vi "Cap_Input.vi"(4 "error in (no error)":errorcluster, 5 "Measured origin x,y":dbl[](array[numeric])=[0.83, 0.79], 6 "Element In":T3, 7 "Outputmode":u16(ring) items=["Get Path", "Make Layout", "Create TRJs"]) -> (0 "error out":errorcluster, 1 "Init Cluster":T6, 2 "TRJs":T4, 3 "Elements Out":T5(array[cluster]))   [LabVIEW 2009]
panel:
  out "output cluster":T1
  in  "Tab Control":enum32{"Main", "Expert", "Output"}(tab)=enum."Output"
  in  "Length of Cap":dbl=3.0
  in  "Radus of Cap":dbl=0.1
  in  "Ab rate":dbl=0.005
  in  "Interval of  laser path":dbl=0.008
  in  "Height to cap":dbl=3.0
  in  "stop":bool
  in  "XY Line Arc Trajectory part 1":T2={"Velocity (units/s)"=2.0, "Acceleration (unts/s2)"=20.0, "Number of times of execution"=1} {"Acceleration (unts/s2)" format="%.6f"; "Velocity (units/s)" format="%.6f"; "Number of times of execution" format="%.6f"}
  in  "Type":i32
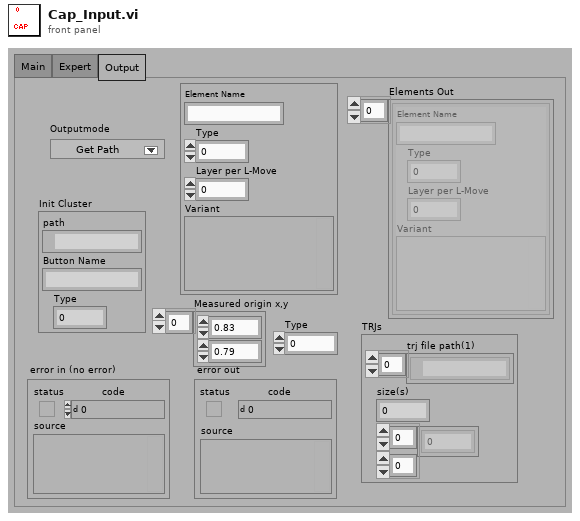
[diagram p1: front panel]
types:
  T1 = cluster{"Length of Cap":dbl, "Height to cap":dbl, "Radus of Cap ":dbl, "Ab rate":dbl, "Interval of  laser path":dbl, "Velocity (units/s)":dbl, "Acceleration (unts/s2)":dbl, "Number of times of execution":i32}
  T2 = cluster{"Velocity (units/s)":dbl, "Acceleration (unts/s2)":dbl, "Number of times of execution":i32}
  T3 = cluster{"Element Name":string, "Type":i32, "Layer per L-Move":i32, "Variant":variant}
  T4 = cluster{"trj file path(1)":path[], "size(s)":i32, dbl[][]}
  T5 = cluster{"Element Name":string, "Type":i32, "Layer per L-Move":i32, "Variant":variant}[]
  T6 = cluster{"path":path, "Button Name":string, "Type":i32}
  T7 = cluster{"Element Name":string, "Value":i32, "Layer per L-Move":i32, "Variant":variant}
  T8 = cluster{"Element Name":string, "Value":i32, "Layer per L-Move":i32, "Variant":variant}[]
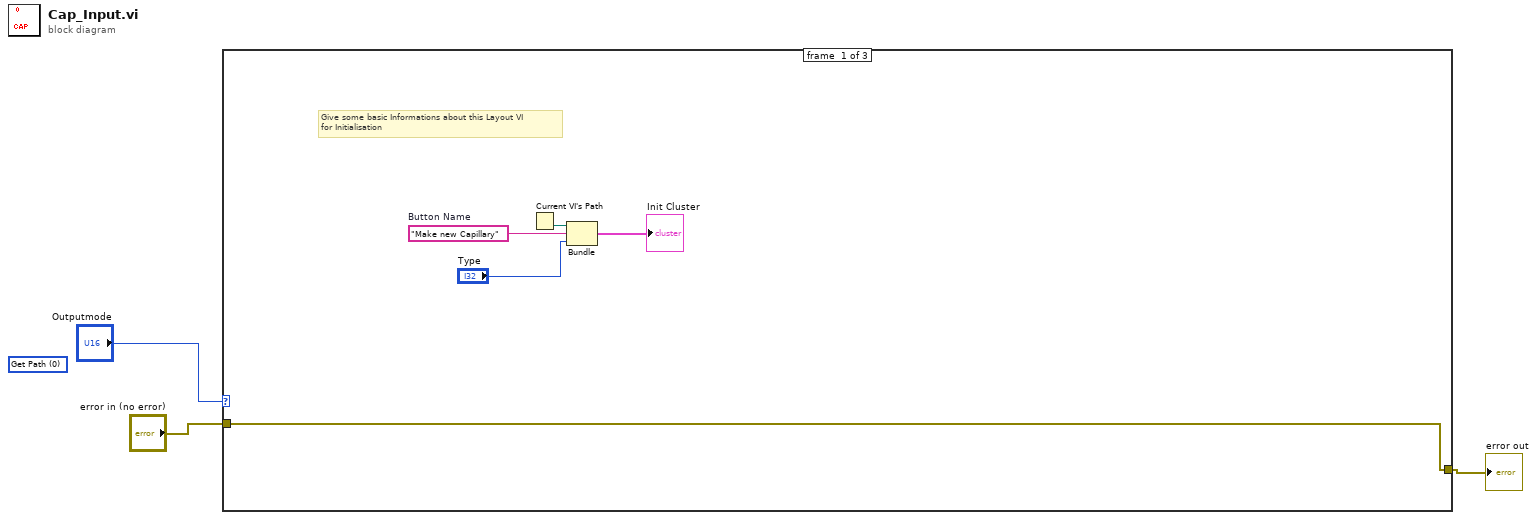
[diagram p0: block diagram]
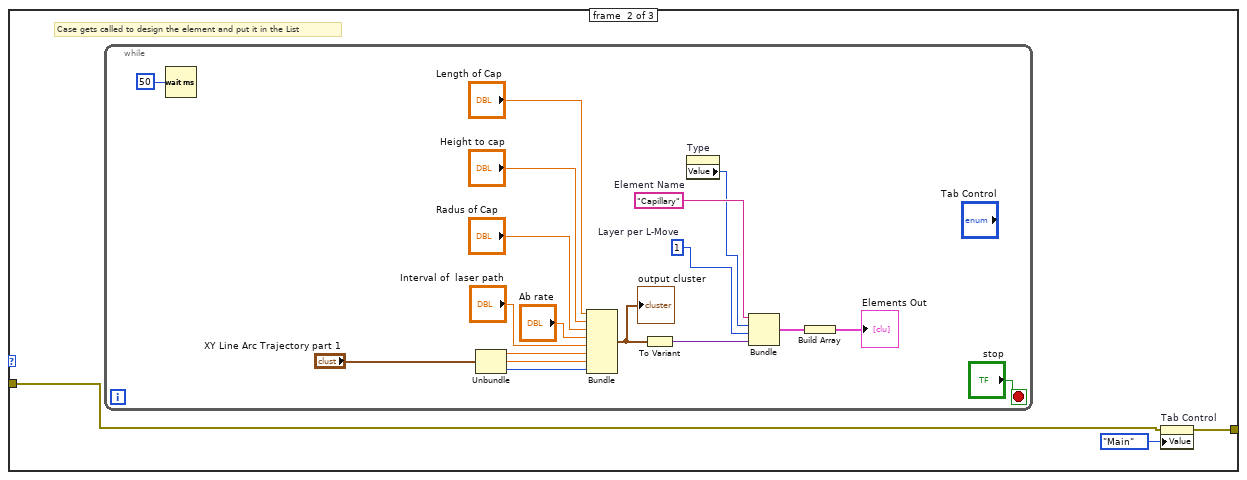
[diagram p2: hidden frame]
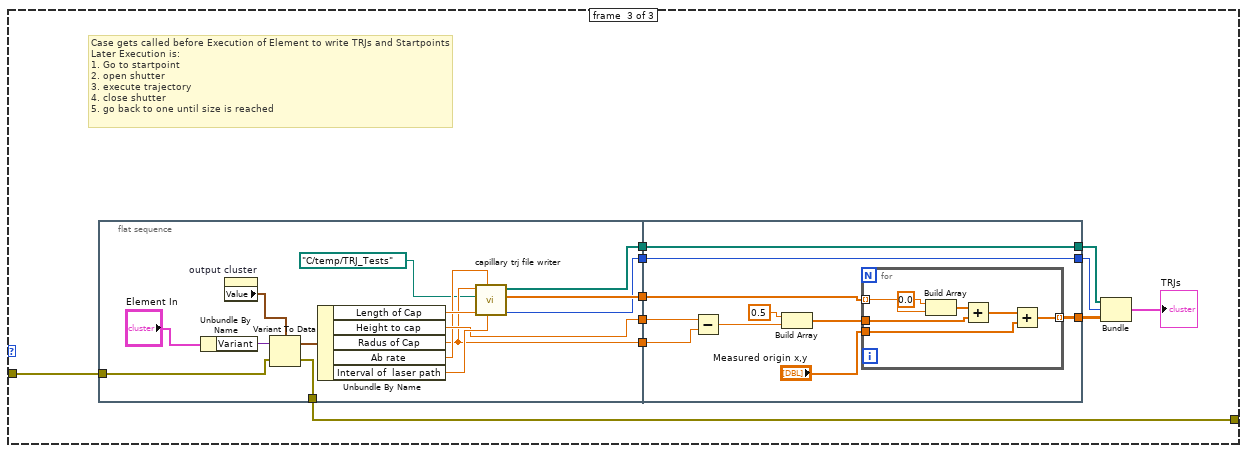
[diagram p3: hidden frame]
diagram:
  (unwired) u16 0 items=["Get Path", "Make Layout", "Create TRJs"] ("Outputmode")
  n1 = case shown="2" "Outputmode" {
    tunnel: "error in (no error)" -> [w8 w10 w31]
    tunnel: [w8 w9 w30] -> w1
    frame #0 {
      w6 = "Make new Capillary"  # Button Name
      # "Give some basic Informations about this Layout VI\nfor Initialisation"
      n2 = Current VI's Path() -> (path=w7:path)
      n3 = Bundle("path"=w7, "Button Name"=w6, "Type"="Type") -> (→"Init Cluster":T6)  [unwired: 1 in]
    }
    frame #1 {
      # "Case gets called to design the element and put it in the List"
      n4 = while {
        stop <- "stop" stop-if-true
        w14 = 1  # Layer per L-Move
        w17 = "Capillary"  # Element Name
        n5 = Wait (ms)(milliseconds to wait=u32 50) -> ()  [unwired: 1 out]
        n6 = Unbundle("XY Line Arc Trajectory part 1") -> ("Velocity (units/s)"=w21:dbl, "Acceleration (unts/s2)"=w20:dbl, "Number of times of execution"=w19:i32)
        n7 = Bundle("Length of Cap"="Length of Cap", "Height to cap"="Height to cap", "Radus of Cap"="Radus of Cap", "Ab rate"="Ab rate", "Interval of  laser path"="Interval of  laser path", "Velocity (units/s)"=w21, "Acceleration (unts/s2)"=w20, "Number of times of execution"=w19) -> (w18:T1)  [unwired: 1 in]
        "output cluster" <- w18
        n8 = To Variant(anything=w18) -> (Variant=w16:variant)
        n9 = property on="Type" class="DigNum (strict)"() -> ("Value"=w12:i32)  [unwired: 2 in, 2 out]
        n10 = Bundle("Element Name"=w17, "Value"=w12, "Layer per L-Move"=w14, "Variant"=w16) -> (w15:T7)  [unwired: 1 in]
        n11 = Build Array(w15) -> (→"Elements Out":T8)
      }
      n12 = property on="Tab Control" class="TabCtl (strict)"(error in=w10, "Value"=enum32{"Main", "Expert", "Output"}."Main" ("Tab Control")) -> (error out=w9:errorcluster)  [unwired: 1 in, 1 out]
    }
    frame #2 {
      # "Case gets called before Execution of Element to write TRJs and Startpoints\nLater Execution is:\n1. Go to startpoint\n2. open shutter\n3. execute trajectory\n4. close shutter\n5. go back to one until size is reached"
      n13 = flat-sequence {
        tunnel: [w55] -> w40
        tunnel: [w54] -> w39
        tunnel: [w53] -> w38
        tunnel: [w47] -> w37
        tunnel: [w45] -> w32
        tunnel: w31 -> [w44]
        tunnel: [w43] -> w30
        tunnel: [w64] -> w35
        tunnel: [w65] -> w36
        tunnel: w40 -> [w65]
        tunnel: w39 -> [w60]
        tunnel: w38 -> [w64]
        tunnel: w37 -> [w59]
        tunnel: [w58] -> w34
        tunnel: w32 -> [w56]
        frame #0 {
          n14 = Unbundle By Name("Element In") -> ("Variant"=w51:variant)
          n15 = property on="output cluster" class="Clust (strict)"() -> ("Value"=w52:T1)  [unwired: 2 in, 2 out]
          n16 = Variant To Data(error in=w44, Variant=w51, type=w52) -> (error out=w43:errorcluster, data=w50:T1)
          n17 = Unbundle By Name(w50) -> ("Length of Cap"=w49:dbl, "Height to cap"=w47:dbl, "Radus of Cap"=w45:dbl, "Ab rate"=w46:dbl, "Interval of  laser path"=w48:dbl)
          n18 = call "capillary trj file writer.vi"("interval between laser path"=w48, "ablation rate"=w46, "length of capillary"=w49, "file (use dialog)"=path "C:/temp/TRJ_Tests", "radus of cap"=w45) -> ("size(s)"=w53:i32, "start point"=w54:dbl[], "trj file path(1)"=w55:path[])  [unwired: 2 out]
        }
        frame #1 {
          n19 = Subtract(x=w59, y=w56) -> (x-y=w61:dbl)
          n20 = Build Array(0.5 ("element"), w61) -> (w63:dbl[])
          n21 = for {
            tunnel: w63 -> [w71]
            tunnel: "Measured origin x,y" -> [w68]
            tunnel: w60 -> [w67] mode=indexing
            tunnel: [w66] -> w58 mode=indexing
            n22 = Build Array(0.0 ("element"), w67) -> (w70:dbl[])
            n23 = Add(x=w70, y=w71) -> (x+y=w72:dbl[])
            n24 = Add(x=w72, y=w68) -> (x+y=w66:dbl[])
          }
        }
      }
      n25 = Bundle("trj file path(1)"=w36, "size(s)"=w35, w34) -> (→"TRJs":T4)  [unwired: 1 in]
    }
  }
  "error out" <- w1
